vi "MGCC_Commun_tran_to_global.vi"() -> ()   [LabVIEW 2016]
uses:
  Global communication.vi
  Model Management/Global_MdlMgmt.vi
panel:
  out "Switch number":dbl
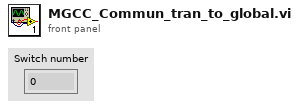
[diagram p1: front panel]
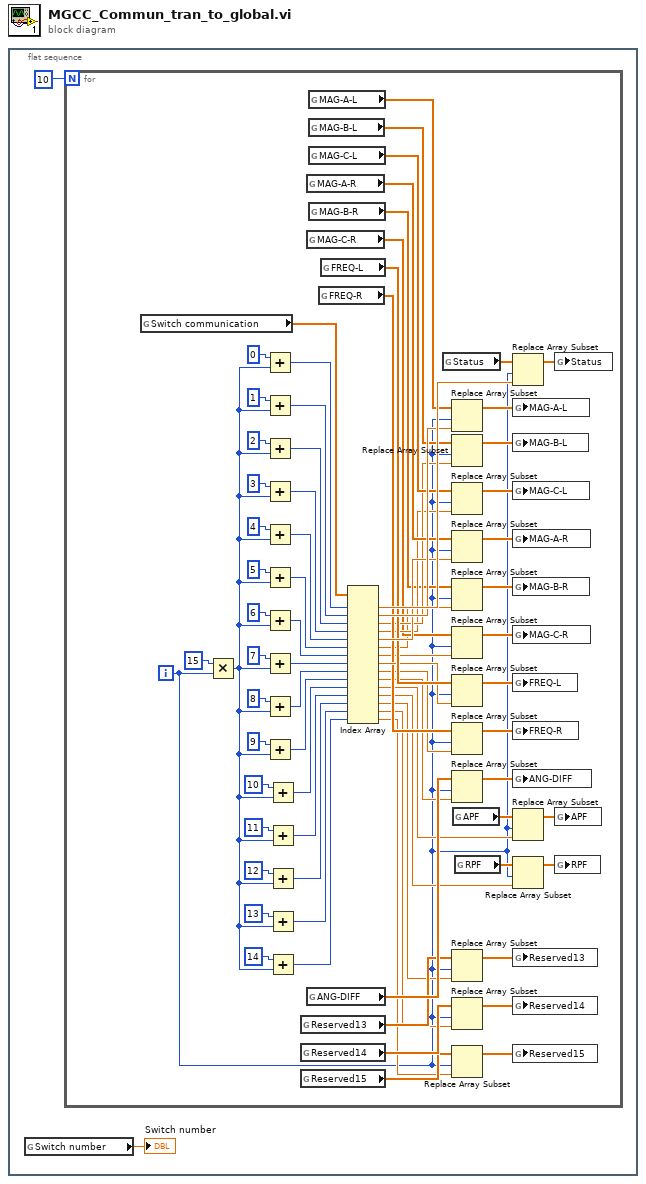
[diagram p0: block diagram]
diagram:
  n1 = flat-sequence {
    frame #0 {
      n2 = global read "Global_MdlMgmt.vi" "Switch number"() -> (→"Switch number":dbl)
      n3 = for {
        N: 10 -> [_]
        i -> [w3]
        n4 = global read "Global communication.vi" "Switch communication"() -> (w18:dbl[])
        n5 = Multiply(x=15, y=w3) -> (x*y=w7:i32)
        n6 = Add(x=0 ("index"), y=w7) -> (x+y=w80:i32)
        n7 = Add(x=1 ("index"), y=w7) -> (x+y=w32:i32)
        n8 = Add(x=2 ("index"), y=w7) -> (x+y=w15:i32)
        n9 = Add(x=3 ("index"), y=w7) -> (x+y=w14:i32)
        n10 = Add(x=4 ("index"), y=w7) -> (x+y=w31:i32)
        n11 = Add(x=5 ("index"), y=w7) -> (x+y=w11:i32)
        n12 = Add(x=6 ("index"), y=w7) -> (x+y=w10:i32)
        n13 = Add(x=7 ("index"), y=w7) -> (x+y=w76:i32)
        n14 = Add(x=8 ("index"), y=w7) -> (x+y=w69:i32)
        n15 = Add(x=9 ("index"), y=w7) -> (x+y=w68:i32)
        n16 = Add(x=10 ("index"), y=w7) -> (x+y=w67:i32)
        n17 = Add(x=11 ("index"), y=w7) -> (x+y=w66:i32)
        n18 = Add(x=12 ("index"), y=w7) -> (x+y=w65:i32)
        n19 = Add(x=13 ("index"), y=w7) -> (x+y=w64:i32)
        n20 = Add(x=14 ("index"), y=w7) -> (x+y=w8:i32)
        n21 = global read "Global communication.vi" "Reserved13"() -> (w37:dbl[])
        n22 = global read "Global communication.vi" "Reserved14"() -> (w34:dbl[])
        n23 = global read "Global communication.vi" "Reserved15"() -> (w5:dbl[])
        n24 = global read "Global communication.vi" "MAG-A-R"() -> (w56:dbl[])
        n25 = global read "Global communication.vi" "MAG-C-R"() -> (w21:dbl[])
        n26 = global read "Global communication.vi" "ANG-DIFF"() -> (w46:dbl[])
        n27 = global read "Global communication.vi" "MAG-A-L"() -> (w59:dbl[])
        n28 = global read "Global communication.vi" "MAG-B-L"() -> (w30:dbl[])
        n29 = global read "Global communication.vi" "MAG-C-L"() -> (w28:dbl[])
        n30 = global read "Global communication.vi" "MAG-B-R"() -> (w22:dbl[])
        n31 = global read "Global communication.vi" "FREQ-R"() -> (w49:dbl[])
        n32 = global read "Global communication.vi" "FREQ-L"() -> (w53:dbl[])
        n33 = Index Array(array=w18, index #1=w80, index #2=w32, index #3=w15, index #4=w14, index #5=w31, index #6=w11, index #7=w10, index #8=w76, index #9=w69, index #10=w68, index #11=w67, index #12=w66, index #13=w65, index #14=w64, index #15=w8) -> (element #1=w60:dbl, element #2=w57:dbl, element #3=w26:dbl, element #4=w25:dbl, element #5=w54:dbl, element #6=w20:dbl, element #7=w19:dbl, element #8=w51:dbl, element #9=w48:dbl, element #10=w45:dbl, element #11=w42:dbl, element #12=w39:dbl, element #13=w36:dbl, element #14=w33:dbl, element #15=w4:dbl)
        n34 = global read "Global communication.vi" "Status"() -> (w62:dbl[])
        n35 = Replace Array Subset(array=w59, new element=w57, index=w3) -> (w58:dbl[])
        n36 = Replace Array Subset(array=w30, new element=w26, index=w3) -> (w29:dbl[])
        n37 = Replace Array Subset(array=w28, new element=w25, index=w3) -> (w27:dbl[])
        n38 = Replace Array Subset(array=w56, new element=w54, index=w3) -> (w55:dbl[])
        n39 = Replace Array Subset(array=w22, new element=w20, index=w3) -> (w24:dbl[])
        n40 = Replace Array Subset(array=w21, new element=w19, index=w3) -> (w23:dbl[])
        n41 = Replace Array Subset(array=w53, new element=w51, index=w3) -> (w52:dbl[])
        n42 = Replace Array Subset(array=w49, new element=w48, index=w3) -> (w50:dbl[])
        n43 = Replace Array Subset(array=w46, new element=w45, index=w3) -> (w47:dbl[])
        n44 = Replace Array Subset(array=w37, new element=w36, index=w3) -> (w38:dbl[])
        n45 = Replace Array Subset(array=w34, new element=w33, index=w3) -> (w35:dbl[])
        n46 = Replace Array Subset(array=w5, new element=w4, index=w3) -> (w6:dbl[])
        n47 = global read "Global communication.vi" "APF"() -> (w43:dbl[])
        n48 = global read "Global communication.vi" "RPF"() -> (w40:dbl[])
        n49 = Replace Array Subset(array=w62, new element=w60, index=w3) -> (w61:dbl[])
        n50 = global write "Global communication.vi" "MAG-A-L"(w58) -> ()
        n51 = global write "Global communication.vi" "MAG-B-L"(w29) -> ()
        n52 = global write "Global communication.vi" "MAG-C-L"(w27) -> ()
        n53 = global write "Global communication.vi" "MAG-A-R"(w55) -> ()
        n54 = global write "Global communication.vi" "MAG-B-R"(w24) -> ()
        n55 = global write "Global communication.vi" "MAG-C-R"(w23) -> ()
        n56 = global write "Global communication.vi" "FREQ-L"(w52) -> ()
        n57 = global write "Global communication.vi" "FREQ-R"(w50) -> ()
        n58 = global write "Global communication.vi" "ANG-DIFF"(w47) -> ()
        n59 = Replace Array Subset(array=w43, new element=w42, index=w3) -> (w44:dbl[])
        n60 = Replace Array Subset(array=w40, new element=w39, index=w3) -> (w41:dbl[])
        n61 = global write "Global communication.vi" "Reserved13"(w38) -> ()
        n62 = global write "Global communication.vi" "Reserved14"(w35) -> ()
        n63 = global write "Global communication.vi" "Reserved15"(w6) -> ()
        n64 = global write "Global communication.vi" "Status"(w61) -> ()
        n65 = global write "Global communication.vi" "APF"(w44) -> ()
        n66 = global write "Global communication.vi" "RPF"(w41) -> ()
      }
    }
  }
